vi "GT_LmtsOn.vi"(3 "limitType":i16(ring) items=["MC_LIMIT_POSITIVE", "MC_LIMIT_NEGATIVE", "BOTH"], 4 "axis":i16, 5 "rtn_In":cluster{"rtn":i16, "Func":string}) -> (1 "axis out":i16, 2 "rtn_Out":cluster{"rtn":i16, "Func":string})   [LabVIEW 2014]
uses:
  VC6/gts.dll
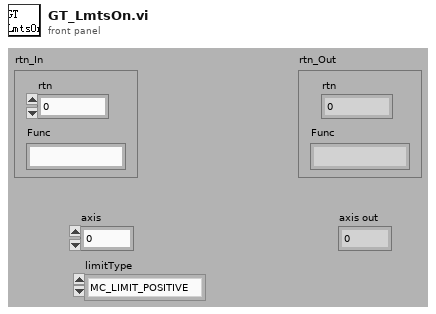
[diagram p1: front panel]
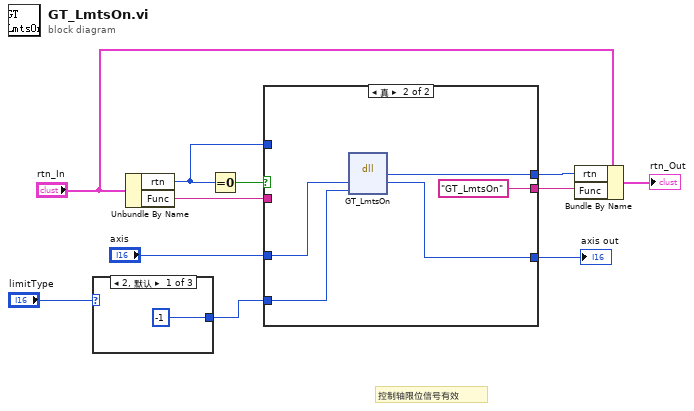
[diagram p0: block diagram]
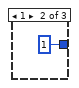
[diagram p2: hidden frame]
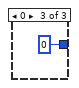
[diagram p3: hidden frame]
diagram:
  # "控制轴限位信号有效"
  n1 = case shown="2, 默认" "limitType" {
    tunnel: [i16 -1 ("limitType") i16 1 ("limitType") i16 0 ("limitType")] -> w2
    frame 2, Default {
    }
    frame 1 {
    }
    frame 0 {
    }
  }
  n2 = Unbundle By Name("rtn_In") -> ("rtn"=w9:i16, "Func"=w10:string)
  n3 = Equal To 0?(x=w9) -> (x = 0?=w11:bool)
  n4 = case shown="真" w11 {
    tunnel: w10 -> [w16 _]
    tunnel: w9 -> [w17 _]
    tunnel: [w17 w22] -> w6
    tunnel: [w16 "GT_LmtsOn" ("Func")] -> w5
    tunnel: "axis" -> [w15 w20]
    tunnel: w2 -> [_ w19]
    tunnel: [w15 w18] -> w1
    frame False {
    }
    frame True {
      n5 = dll-call lib="PTH2Fabs DNewGTS AC-800LWin7版源程序-20170926gts85VC6gts.dll" fn="GT_LmtsOn"("axis"=w20, "limitType"=w19) -> ("rtn"=w22:i16, "axis"=w18:i16)  [unwired: 4 in, 2 out]
    }
  }
  "axis out" <- w1
  n6 = Bundle By Name(cluster="rtn_In", "rtn"=w6, "Func"=w5) -> (→"rtn_Out":cluster{"rtn":i16, "Func":string})
